vi "queue-1.vi"() -> ()   [LabVIEW 2020]
uses:
  <vilib>/Utility/error.llb/DialogType.ctl
panel:
  out "# elements in queue":i32
  in  "milliseconds to wait":u32
  out "Waveform Chart 2":i32(graph)
  out "Waveform Chart":i32(graph)
  in  "stop":bool
  out "x-y*floor(x/y)":i32
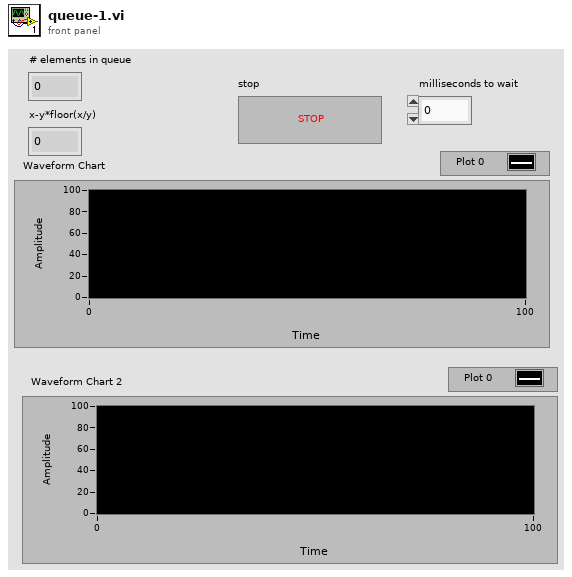
[diagram p1: front panel]
types:
  T1 = typedef "DialogType.ctl" = u16
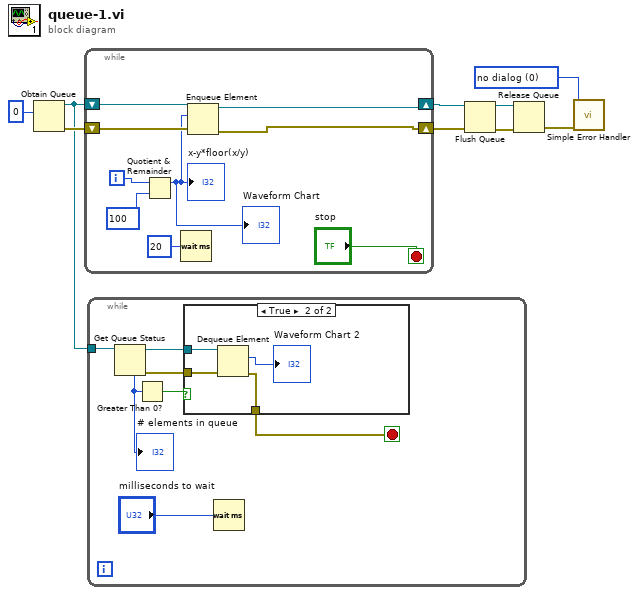
[diagram p0: block diagram]
diagram:
  w2 = T1 0 items=["no dialog", "OK message", "continue or stop message", "OK message + warnings", "continue/stop + warnings"] ("type of dialog (OK msg:1)")
  n1 = Obtain Queue(element data type=0) -> (queue out=w1:refnum<queue>, error out=w8:errorcluster)  [unwired: 4 in, 1 out]
  n2 = while {
    shift-right: [w11] -> w6
    shift-left: w1 -> [w14]
    shift-right: [w10] -> w7
    shift-left: w8 -> [w13]
    i -> [w18]
    stop <- "stop" stop-if-true
    n3 = Quotient & Remainder(x=w18, y=100) -> (x-y*floor(x/y)=w12:i32)  [unwired: 1 out]
    "x-y*floor(x/y)" <- w12
    "Waveform Chart" <- w12
    n4 = Wait (ms)(milliseconds to wait=u32 20) -> ()  [unwired: 1 out]
    n5 = Enqueue Element(queue=w14, element=w12, error in (no error)=w13) -> (queue out=w11:refnum<queue>, error out=w10:errorcluster)  [unwired: 1 in, 1 out]
  }
  n6 = while {
    tunnel: w1 -> [w24]
    stop <- w19 stop-if-true
    n7 = Get Queue Status(queue=w24) -> (queue out=w21:refnum<queue>, error out=w20:errorcluster, # elements in queue=w23:i32)  [unwired: 2 in, 5 out]
    "# elements in queue" <- w23
    n8 = Greater Than 0?(x=w23) -> (x > 0?=w22:bool)
    n9 = case shown="True" w22 {
      tunnel: w21 -> [_ w30]
      tunnel: w20 -> [w26 w29]
      tunnel: [w26 w27] -> w19
      frame False {
      }
      frame True {
        n10 = Dequeue Element(queue=w30, error in (no error)=w29) -> (element=→"Waveform Chart 2":i32, error out=w27:errorcluster)  [unwired: 1 in, 2 out]
      }
    }
    n11 = Wait (ms)(milliseconds to wait="milliseconds to wait") -> ()  [unwired: 1 out]
  }
  n12 = Flush Queue(queue=w6, error in (no error)=w7) -> (queue out=w4:refnum<queue>, error out=w5:errorcluster)  [unwired: 1 out]
  n13 = Release Queue(queue=w4, error in (no error)=w5) -> (error out=w3:errorcluster)  [unwired: 1 in, 2 out]
  n14 = call <vilib>:"Simple Error Handler.vi"("type of dialog (OK msg:1)"=w2, "error in (no error)"=w3) -> ()  [unwired: 3 in, 5 out]
